vi "CH_LM Config Trigger Level.vi"(0 "Meter Index":i32, 2 "Trigger Level (5%)":dbl=5.0 format="%#.3g", 5 "error in (no error)":errorcluster, 7 "Timeout / ms (3000)":i32=3000, 8 "Action (query)":bool, 9 "Lock Timeout / ms (1000)":i32=1000) -> (11 "Lock timed out":bool, 14 "Meter Index":i32, 16 "Trigger Level / %":dbl format="%#.3g", 19 "error out":errorcluster)   [LabVIEW 2012, in "CH_LM.lvlib"]
doc: "This command will set/query the trigger level expressed as a percentage of full scale capability for pyroelectric probes. (TOP only)\n\n<B>Note:</B> To be used with Internal Trigger Source."
uses:
  CH_LM.lvlib
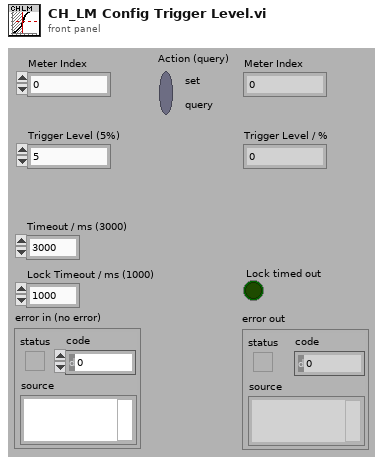
[diagram p1: front panel]
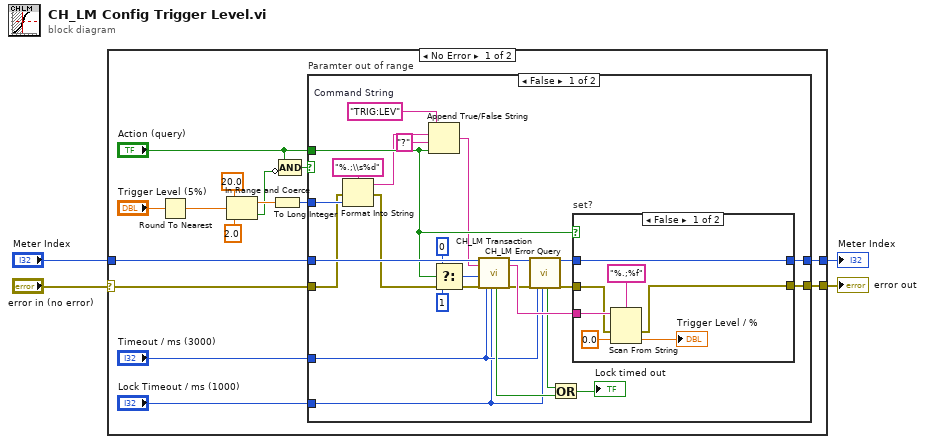
[diagram p0: block diagram]
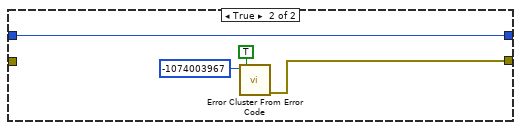
[diagram p3: hidden frame]
diagram:
  n1 = case shown="No Error" "error in (no error)" {
    selector: "error in (no error)" -> [w19 w59]
    tunnel: [w17 w59] -> w4
    tunnel: "Meter Index" -> [w18 w58]
    tunnel: [w16 w58] -> w1
    frame No Error {
      n2 = Round To Nearest(number="Trigger Level (5%)") -> (nearest integer value=w6:dbl)
      n3 = In Range and Coerce(upper limit=20.0, x=w6, lower limit=2.0) -> (coerced(x)=w12:dbl, In Range?=w9:bool)
      n4 = To Long Integer(number=w12) -> (32bit integer=w5:i32)
      n5 = Compound Arithmetic op=AND("Action (query)", invert w9) -> (w7:bool)
      n6 = case "Paramter out of range" shown="False" w7 {
        tunnel: w19 -> [w23 _]
        tunnel: w18 -> [w44 w57]
        tunnel: [w41 w55] -> w17
        tunnel: [w35 w57] -> w16
        tunnel: "Timeout / ms (3000)" -> [w27 _]
        tunnel: "Lock Timeout / ms (1000)" -> [w26 _]
        tunnel: w5 -> [w24 _]
        tunnel: "Action (query)" -> [w25 _]
        frame False {
          w43 = "TRIG:LEV"  # Command String
          n7 = Format Into String(format string="%.;\\s%d", error in=w23, w24) -> (resulting string=w20:string, error out=w22:errorcluster)  [unwired: 1 in]
          n8 = Append True/False String(1:w25, 2:"?" ("true string"), 3:w20, 4:w43) -> (0:w21:string)
          n9 = Select(t=0, s=w25, f=1 ("NofStrings (-1:all)")) -> (s? t:f=w37:i32)
          n10 = call "CH_LM Transaction.vi"("Meter Index"=w44, "Command String"=w21, "NofStrings (-1:all)"=w37, "error in (no error)"=w22, "Timeout / ms (3000)"=w27, "Lock Timeout / ms (1000)"=w26) -> ("Lock timed out"=w29:bool, "Meter Index"=w34:i32, "Response"=w42:string, "error out"=w32:errorcluster)  [unwired: 10 out]
          n11 = call "CH_LM Error Query.vi"("Meter Index"=w34, "error in (no error)"=w32, "Timeout / ms (3000)"=w27, "Lock Timeout / ms (1000)"=w26) -> ("Lock timed out"=w30:bool, "Meter Index"=w33:i32, "error out"=w31:errorcluster)  [unwired: 13 out]
          n12 = Or(x=w30, y=w29) -> (x .or. y?=→"Lock timed out":bool)
          n13 = case "set?" shown="False" w25 {
            tunnel: w42 -> [w51 _]
            tunnel: w31 -> [w50 w53]
            tunnel: [w49 w53] -> w41
            tunnel: w33 -> [w46 w52]
            tunnel: [w46 w52] -> w35
            frame False {
              n14 = Scan From String(format string="%.;%f", input string=w51, error in=w50, default 1=0.0 ("default value 1")) -> (error out=w49:errorcluster, output 1=→"Trigger Level / %":dbl)  [unwired: 1 in, 2 out]
            }
            frame True {
            }
          }
        }
        frame True {
          n15 = call <vilib>:"Error Cluster From Error Code.vi"("show call chain? (False)"=TRUE, "error code (0)"=-1074003967) -> ("error out"=w55:errorcluster)  [unwired: 1 in, 6 out]
        }
      }
    }
    frame Error {
    }
  }
  "error out" <- w4
  "Meter Index" <- w1
